vi "readFromXML.vi"(8 "error in (no error)":errorcluster, 10 "XML in":string, 11 "GuideTargetAbsorbOffset in":refnum<class "GuideTargetAbsorbOffset.lvclass">) -> (0 "error out":errorcluster, 3 "GuideTargetAbsorbOffset out":refnum<class "GuideTargetAbsorbOffset.lvclass">)   [LabVIEW 2014, in "TCSDataDefinitions.lvlib" / "TCSCommand.lvlib" / "OffsetCommands.lvlib" / "GuideTargetAbsorbOffset.lvclass"]
uses:
  GuideTargetAbsorbOffset.lvclass
  AbsorbOffset/AbsorbOffset.lvclass
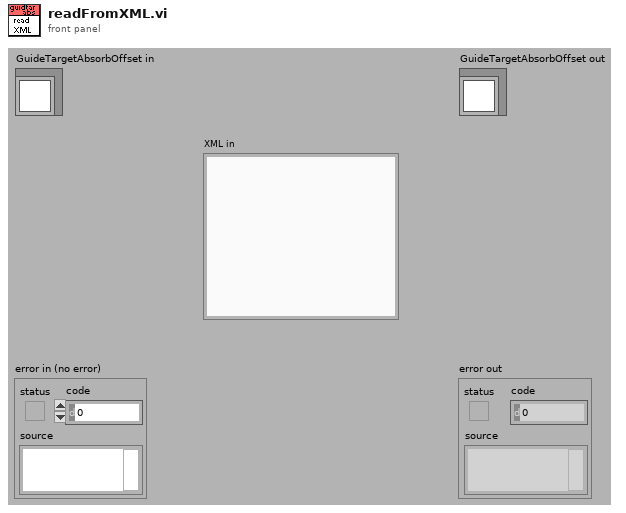
[diagram p1: front panel]
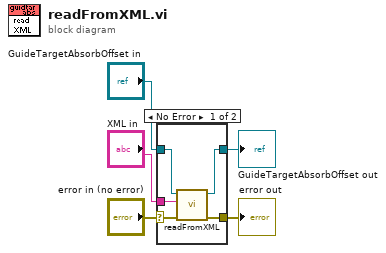
[diagram p0: block diagram]
diagram:
  n1 = case shown="No Error" "error in (no error)" {
    selector: "error in (no error)" -> [w7 w12]
    tunnel: [w6 w12] -> w4
    tunnel: [w8 w11] -> w2
    tunnel: "GuideTargetAbsorbOffset in" -> [w9 w11]
    tunnel: "XML in" -> [w10 _]
    frame No Error {
      n2 = call-parent "readFromXML.vi"("error in (no error)"=w7, "XML in"=w10, "AbsorbOffset in"=w9) -> ("error out"=w6:errorcluster, "AbsorbOffset out"=w8:refnum<class "GuideTargetAbsorbOffset.lvclass">)  [unwired: 7 out]
    }
    frame Error {
    }
  }
  "error out" <- w4
  "GuideTargetAbsorbOffset out" <- w2
